vi "updateStatistics.vi"(10 "Temperature":dbl, 11 "StatisticsData in":T1) -> (3 "StatisticsData out":T1)   [LabVIEW 2020, in "StatisticsDisplay.lvclass"]
uses:
  StatisticsDisplay.lvclass
  StatisticsData.ctl
  StatisticsDisplay.lvclass/StatisticsDisplay.ctl
panel:
  # "Connector Pane"
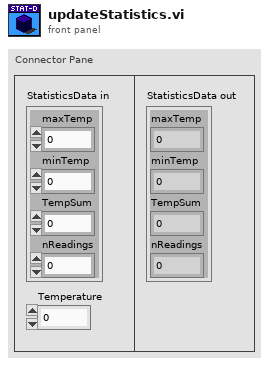
[diagram p1: front panel]
types:
  T1 = typedef "StatisticsDisplay.lvclass/StatisticsData.ctl" = cluster{"maxTemp":dbl, "minTemp":dbl, "TempSum":dbl, "nReadings":i32}
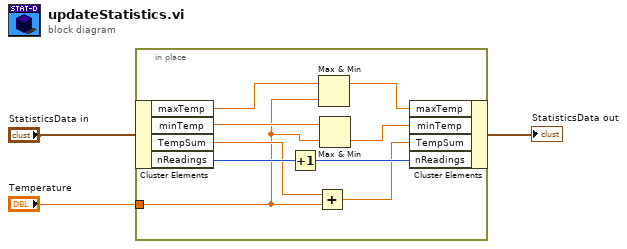
[diagram p0: block diagram]
diagram:
  n1 = in-place {
    in-place-border: "Temperature" -> [w4]
    n2 = in-place-cluster #1("StatisticsData in") -> ("maxTemp"=w8:dbl, "minTemp"=w5:dbl, "TempSum"=w10:dbl, "nReadings"=w12:i32)
    n3 = Increment(x=w12) -> (x+1=w11:i32)
    n4 = Add(x=w10, y=w4) -> (x+y=w9:dbl)
    n5 = Max & Min(x=w8, y=w4) -> (max(x,y)=w7:dbl)  [unwired: 1 out]
    n6 = Max & Min(x=w5, y=w4) -> (min(x,y)=w6:dbl)  [unwired: 1 out]
    n7 = in-place-cluster #1("maxTemp"=w7, "minTemp"=w6, "TempSum"=w9, "nReadings"=w11) -> (→"StatisticsData out":T1)
  }
